vi "Process.vi"(8 "error in (no error)":errorcluster, 10 "Results Notifier":refnum<notifier>, 11 "WriteCommand in":refnum<class "WriteCommand.lvclass">) -> (0 "error out":errorcluster, 3 "WriteCommand out":refnum<class "WriteCommand.lvclass">)   [LabVIEW 2023, in "HAF.lvlib" / "WriteCommand.lvclass"]
doc: "Processes the Write Command against the specified Driver for the Command.\n\nThe Driver will ensure it is initialised and process the Command Settings; it is responsible for interacting with the Instrument.\n\nAny Results Notifier passed is ignored by a Write Command, because no result is processed. It may be used by a Read Command."
uses:
  WriteCommand.lvclass
  WriteCommand.lvclass/WriteCommand.ctl
  Driver/Driver.lvclass
  Executable/Executable.lvclass
  \\Mac\Home/Documents/LabVIEW Data/ProjectTemplates/Source/HAF/WriteCommand/WriteCommand.lvclass
  \\Mac\Home/Documents/LabVIEW Data/ProjectTemplates/Source/HAF/Executable/Executable.lvclass
  ReadCommand/ReadCommand.lvclass
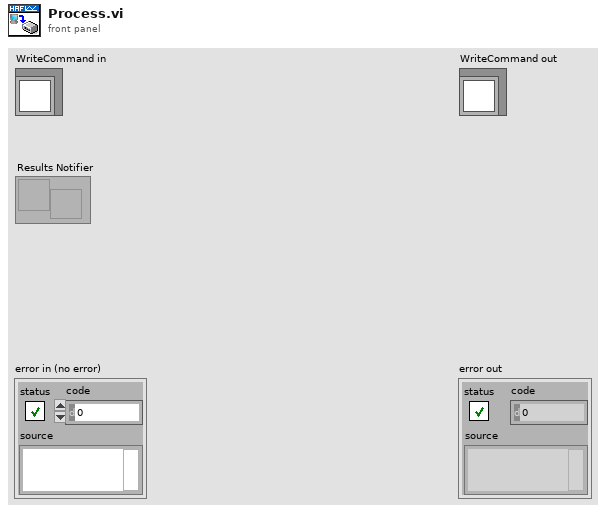
[diagram p1: front panel]
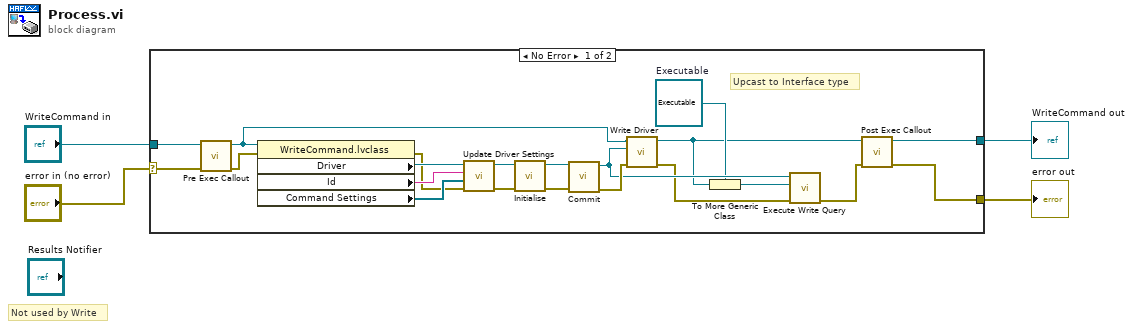
[diagram p0: block diagram]
diagram:
  # "Not used by Write"
  n1 = case shown="No Error" "error in (no error)" {
    selector: "error in (no error)" -> [w24 w27]
    tunnel: [w5 w27] -> w3
    tunnel: [w6 w26] -> w1
    tunnel: "WriteCommand in" -> [w25 w26]
    frame No Error {
      w10 = refnum<class "Executable.lvclass"> refnum  # Executable
      # "Upcast to Interface type"
      n2 = call-dynamic "Pre Exec Callout.vi"("error in (no error)"=w24, "WriteCommand in"=w25) -> ("error out"=w23:errorcluster, "WriteCommand out"=w14:refnum<class "WriteCommand.lvclass">)  [unwired: 8 in]
      n3 = property class="WriteCommand.lvclass"(reference=w14, error in=w23) -> (error out=w19:errorcluster, "Driver"=w22:refnum<class "Driver.lvclass">, "Id"=w21:string, "Command Settings"=w20:refnum<class "CommandSetting.lvclass">[])  [unwired: 1 out]
      n4 = call-dynamic "Update Driver Settings.vi"("error in (no error)"=w19, "Command Settings"=w20, "Command Id"=w21, "Driver in"=w22) -> ("error out"=w17:errorcluster, "Driver out"=w18:refnum<class "Driver.lvclass">)  [unwired: 4 in, 2 out]
      n5 = call-dynamic "Initialise.vi"("error in (no error)"=w17, "Driver in"=w18) -> ("error out"=w15:errorcluster, "Driver out"=w16:refnum<class "Driver.lvclass">)  [unwired: 8 in]
      n6 = call-dynamic "Commit.vi"("error in (no error)"=w15, "Driver in"=w16) -> ("error out"=w13:errorcluster, "Driver out"=w12:refnum<class "Driver.lvclass">)  [unwired: 8 in]
      n7 = call-dynamic "Write Driver.vi"("error in (no error)"=w13, "HAF:Driver.lvclass"=w12, "WriteCommand in"=w14) -> ("error out"=w11:errorcluster, "WriteCommand out"=w8:refnum<class "WriteCommand.lvclass">)  [unwired: 7 in]
      n8 = To More Generic Class(target class=w10, reference=w8) -> (generic class reference=w9:refnum<class "Executable.lvclass">)
      n9 = call-dynamic "Execute Write Query.vi"("error in (no error)"=w11, "Executable In"=w9, "Driver in"=w12) -> ("error out"=w7:errorcluster)  [unwired: 6 in, 2 out]
      n10 = call-dynamic "Post Exec Callout.vi"("error in (no error)"=w7, "WriteCommand in"=w8) -> ("error out"=w5:errorcluster, "WriteCommand out"=w6:refnum<class "WriteCommand.lvclass">)  [unwired: 8 in]
    }
    frame Error {
    }
  }
  "error out" <- w3
  "WriteCommand out" <- w1
